vi "user initialization.vi"(8 "error in":errorcluster, 10 "configuration in":refnum<class "control module configuration.lvclass">, 11 "fixed channel runtime in":refnum<class "BuckBoost runtime.lvclass">) -> (0 "error out":errorcluster, 3 "fixed channel runtime out":refnum<class "BuckBoost runtime.lvclass">)   [LabVIEW 2017, in "BuckBoost runtime.lvclass"]
uses:
  BuckBoost runtime.lvclass
  <vilib>/NI/DCAF/Tag Editor Core/control module/configuration/control module configuration.lvclass
  configuration/BuckBoost configuration.lvclass
  C:/Program Files (x86)/National Instruments/LabVIEW 2017/vi.lib/NI/DCAF/Tag Editor Core/control module/configuration/control module configuration.lvclass
  <vilib>/userdefined/High Color/nirio_resource_hc.ctl
  <vilib>/NI/DCAF/addons/InstructionFrameworkSupport/FPGA_FGV_action.ctl
  configuration/BuckBoost configuration.lvclass/BuckBoost configuration.ctl
  BuckBoost runtime.lvclass/BuckBoost runtime.ctl
  configuration/Read numOfInterleaves.vi
  configuration/Read rampRate.vi
  configuration/Read gains.vi
  configuration/Read modulationConfig.vi
  <instrlib>/_niInstr/FIFO Register Bus/v1/Host/niInstr FIFO Register Bus v1 Host.lvclass
  C:/Program Files (x86)/National Instruments/LabVIEW 2017/instr.lib/_niInstr/Instruction Framework/v1/Host/Instruction Target/niInstr Instruction Target v1 Host.lvclass
  <vilib>/NI/DCAF/Tag Editor Core/control module/runtime/control module runtime.lvclass
  <instrlib>/_niInstr/Instruction Framework/v1/Host/Subsystem Map/niInstr Subsystem Map v1 Host.lvclass
  <vilib>/NI/PowerElectronicsControl/Buck-Boost/RealTime/BuckBoostInterface.lvlib
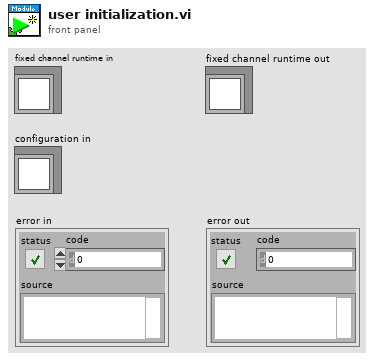
[diagram p1: front panel]
types:
  T1 = typedef "FPGA_FGV_action.ctl" = enum16{"get FPGA", "set FPGA", "Close"}
  T2 = typedef "nirio_resource_hc.ctl" = tag
  T3 = typedef "niFpgaPID_PIGains.ctl" = cluster{"proportional gain":sgl, "integral gain":sgl}
  T4 = typedef "BuckBoostInterface.lvlib/modulationConfig.ctl" = cluster{"SwitchingSpeed":dbl, "Deadband":dbl, "modulationRate":dbl}
  T5 = typedef "BuckBoostInterface.lvlib/Interface.ctl" = cluster{"instruction target":refnum<class "niInstr Instruction Target v1 Host.lvclass">, "BuckBoostContext":refnum<class "niInstr Instruction Framework Context v1 Host.lvclass">}
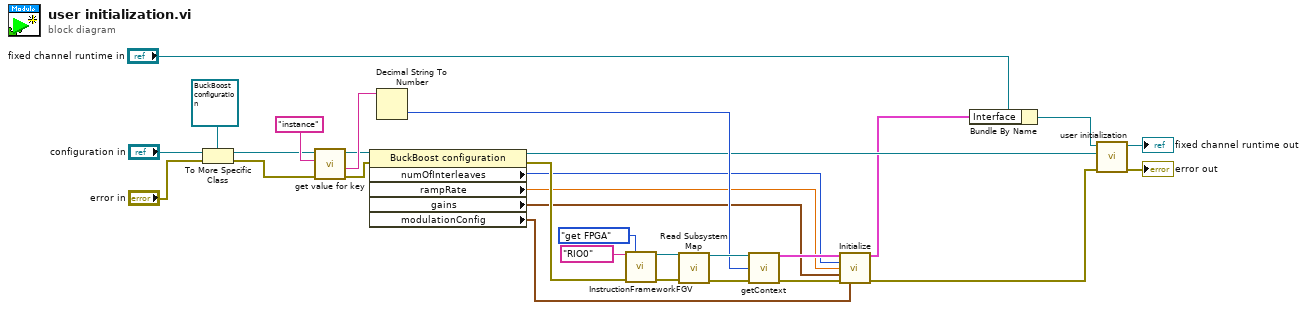
[diagram p0: block diagram]
diagram:
  n1 = To More Specific Class(target class=refnum<class "BuckBoost configuration.lvclass"> refnum ("BuckBoost configuration"), reference="configuration in", error in="error in") -> (specific class reference=w24:refnum<class "BuckBoost configuration.lvclass">, error out=w23:errorcluster)
  n2 = call-dynamic "get value for key.vi"("error in"=w23, "key"="instance", "fixed channel configuration in"=w24) -> ("error out"=w11:errorcluster, "value"=w22:string, "fixed channel configuration out"=w12:refnum<class "BuckBoost configuration.lvclass">)  [unwired: 6 in]
  n3 = property class="BuckBoost configuration"(reference=w12, error in=w11) -> (reference out=w5:refnum<class "BuckBoost configuration.lvclass">, error out=w10:errorcluster, "numOfInterleaves"=w9:u8, "rampRate"=w8:sgl, "gains"=w7:T3, "modulationConfig"=w6:T4)
  n4 = Decimal String To Number(string=w22) -> (number=w15:i32)  [unwired: 2 in, 1 out]
  n5 = call <vilib>:"InstructionFrameworkFGV.vi"("RIO resource"=T2 "RIO0", "Action"=FPGA_FGV_action."get FPGA", "error in"=w10) -> ("session out"=w18:refnum<class "niInstr FIFO Register Bus v1 Host.lvclass">, "error out"=w19:errorcluster)  [unwired: 10 in, 1 out]
  n6 = call <instrlib>:"Read Subsystem Map.vi"("instruction target in"=w18, "error in"=w19) -> ("instruction target out"=w17:refnum<class "niInstr FIFO Register Bus v1 Host.lvclass">, "error out"=w16:errorcluster)  [unwired: 11 in, 1 out]
  n7 = call <vilib>:"getContext.vi"("instruction target in"=w17, "instance"=w15, "error in"=w16) -> ("Interface"=w14:T5, "error out"=w13:errorcluster)  [unwired: 11 in]
  n8 = call <vilib>:"Initialize.vi"("Interface in"=w14, "numOfInterleaves"=w9, "rampRate"=w8, "gains"=w7, "error in"=w13, "modulationConfig"=w6) -> ("Interface out"=w1:T5, "error out"=w4:errorcluster)  [unwired: 8 in]
  n9 = Bundle By Name(cluster="fixed channel runtime in", "Interface"=w1) -> (w2:refnum<class "BuckBoost runtime.lvclass">)
  n10 = call-parent "user initialization.vi"("error in"=w4, "configuration in"=w5, "fixed channel runtime in"=w2) -> ("error out"=→"error out":errorcluster, "fixed channel runtime out"=→"fixed channel runtime out":refnum<class "BuckBoost runtime.lvclass">)  [unwired: 7 in]
